vi "test5-ChainNodeBroadcast.vi"(8 "error in (no error)":errorcluster, 11 "TestCase in":refnum<class "testcase-CSMChainMode.lvclass">) -> (0 "error out":errorcluster, 3 "TestCase out":refnum<class "testcase-CSMChainMode.lvclass">)   [LabVIEW 2017, in "testcase-CSMChainMode.lvclass"]
uses:
  testcase-CSMChainMode.lvclass
  b9a68168-9423-447a-be7f-8ac0ebad77aa.vi
  a50093c0-808a-49cf-b933-7f76f8d4e341.vi
  src/user.lib/_NEVSTOP/Communicable State Machine(CSM)/AdvanceAPI/CSM - Get Module Attribute.vi
  <vilib>/addons/_JKI Toolkits/VI Tester/TestCase.llb/TestCase.lvclass
  src/user.lib/_NEVSTOP/Communicable State Machine(CSM)/Communicable State Machine.lvlib
  C:/Program Files (x86)/National Instruments/LabVIEW 2017/vi.lib/addons/_JKI Toolkits/VI Tester/TestCase.llb/TestCase.lvclass
panel:
  out "LoopCount":i32
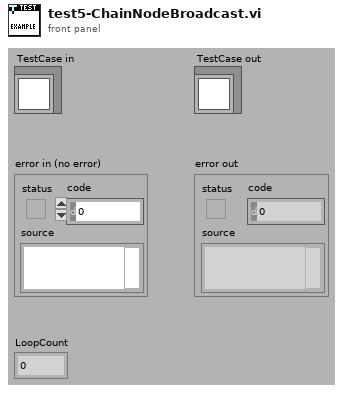
[diagram p1: front panel]
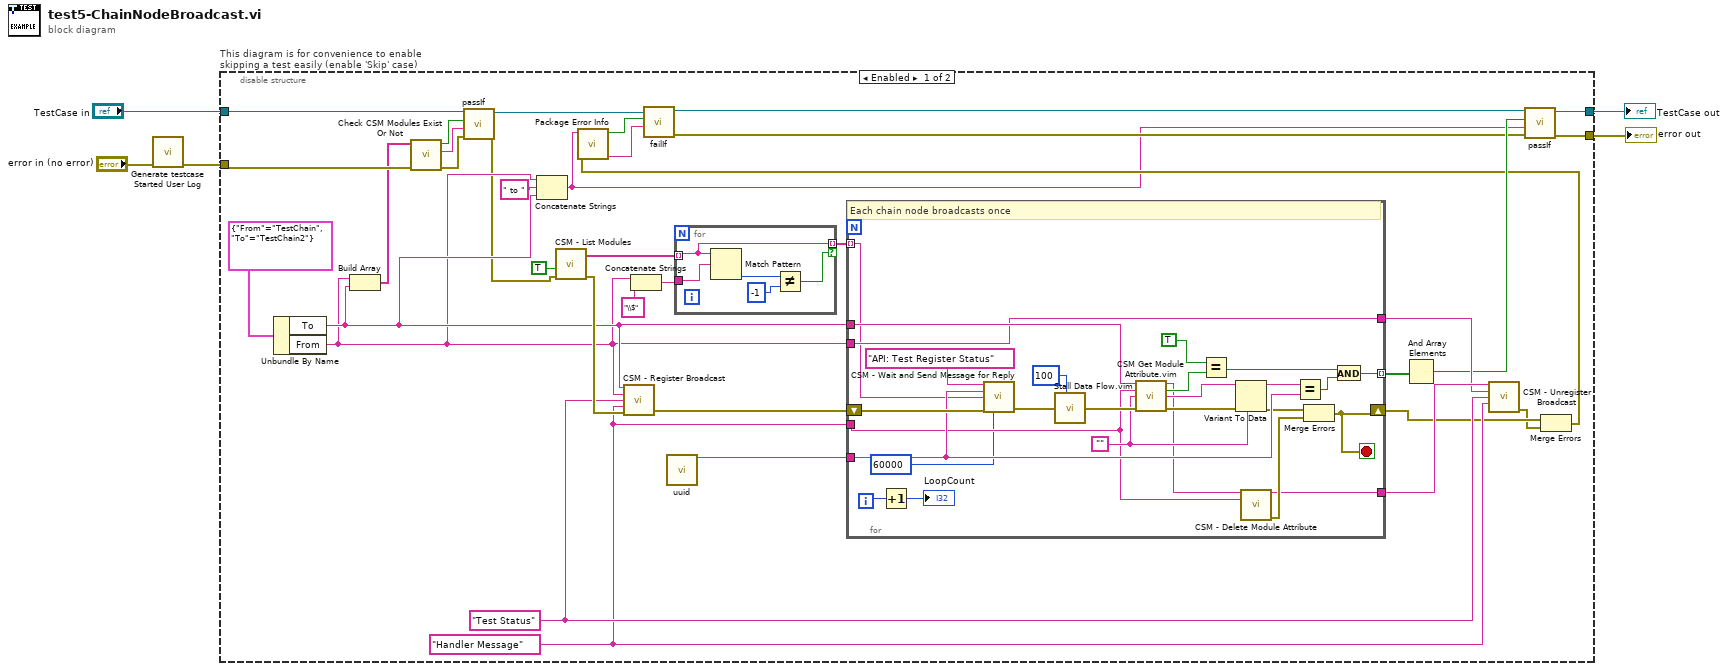
[diagram p0: block diagram]
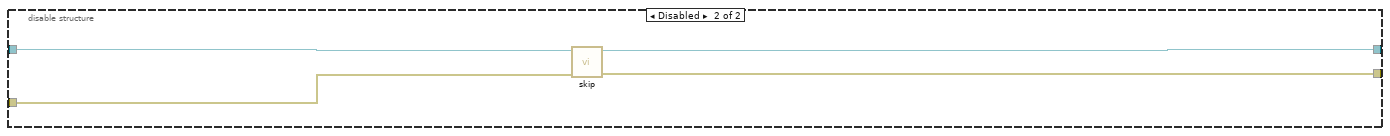
[diagram p2: hidden frame]
diagram:
  n1 = call "Generate testcase Started User Log.vi"("Error In"="error in (no error)") -> ("error out"=w1:errorcluster)  [unwired: 10 in]
  n2 = disable-structure "This diagram is for convenience to enable skipping a test easily (enable 'Skip' case)" shown="Enabled" {
    disable-tunnel: "TestCase in" -> [w15 w77]
    disable-tunnel: [w25 w75] -> w2
    disable-tunnel: [w24 w76] -> w4
    disable-tunnel: w1 -> [w13 w74]
    frame Enabled {
      w31 = "Handler Message" ("API (If \"\", Same as Trigger)")
      w32 = "Test Status" ("Trigger")
      n3 = Unbundle By Name(cluster{"From":string, "To":string} {"From"="TestChain", "To"="TestChain2"} ("Cluster")) -> ("To"=w11:string, "From"=w10:string)
      n4 = Build Array(w10, w11) -> (w12:string[])
      n5 = call "Check CSM Modules Exist Or Not.vi"("error in"=w13, "CSM names in"=w12) -> ("error out"=w20:errorcluster, "Debug string"=w21:string, "All Modules Exist?"=w22:bool)  [unwired: 7 in]
      n6 = call-dynamic "passIf.vi"("error in (no error)"=w20, "message (\"\")"=w21, "pass"=w22, "TestCase in"=w15) -> ("error out"=w9:errorcluster, "TestCase out"=w16:refnum<class "testcase-CSMChainMode.lvclass">)  [unwired: 6 in]
      n7 = Concatenate Strings(w10, " to " ("string"), w11) -> (w6:string)
      n8 = call "CSM - List Modules.vi"("Error In"=w9, "With Nodes? (F)"=TRUE) -> ("error out"=w34:errorcluster, "Module Names"=w37:string[])  [unwired: 8 in]
      n9 = call "CSM - Register Broadcast.vi"("CSM Name(Empty for Broadcast Event)"=w11, "Source CSM Name (* as Default)"=w10, "Trigger"=w32, "API (If \"\", Same as Trigger)"=w31, "Error In"=w34) -> ("error out"=w36:errorcluster)  [unwired: 9 in, 1 out]
      n10 = Concatenate Strings(w10, "\\$" ("string")) -> (w39:string)
      n11 = call "uuid.vi"() -> ("UUID"=w35:string)  [unwired: 11 in]
      n12 = for {
        tunnel: w37 -> [w71] mode=indexing
        tunnel: [w71] -> w33 mode=indexing if=w70
        tunnel: w39 -> [w69]
        n13 = Match Pattern(string=w71, regular expression=w69) -> (offset past match=w73:i32)  [unwired: 1 in, 3 out]
        n14 = Not Equal?(x=w73, y=-1) -> (x != y?=w70:bool)
      }
      n15 = for {
        tunnel: w35 -> [w54]
        tunnel: w33 -> [w44] mode=indexing
        tunnel: w11 -> [w61]
        tunnel: w31 -> [w50]
        shift-right: [w43] -> w28
        shift-left: w36 -> [w67]
        tunnel: w10 -> [w45]
        tunnel: [w47] -> w30
        tunnel: [w45] -> w29
        tunnel: [w46] -> w26 mode=indexing
        i -> [w66]
        stop <- w43 stop-if-true
        w56 = ""
        # "Each chain node broadcasts once"
        n16 = Increment(x=w66) -> (x+1=→"LoopCount":i32)
        n17 = call "CSM - Wait and Send Message for Reply.vi"("State"="API: Test Register Status", "Arguments (\"\")"=w54, "Target Module"=w44, "Error In (No Error)"=w67, "Response Timeout (-2 Using Global Settings)"=60000) -> ("error out"=w64:errorcluster)  [unwired: 7 in, 3 out]
        n18 = call "Stall Data Flow.vim"("value in"=w64, "milliseconds to wait"=u32 100) -> ("value out"=w62:errorcluster)  [unwired: 1 out]
        n19 = call "CSM Get Module Attribute.vim"("CSM Name"=w61, "Attribute"=w50, "Default Value (Empty Variant)"=w56, "Error In"=w62) -> ("CSM Name (Dup)"=w51:string, "Found"=w59:bool, "Value"=w57:string, "error out"=w58:errorcluster)  [unwired: 7 in, 1 out]
        n20 = Equal?(x=TRUE, y=w59) -> (x = y?=w52:bool)
        n21 = Variant To Data(error in=w58, type=w56, Variant=w57) -> (data=w55:string, error out=w49:errorcluster)
        n22 = call "CSM - Delete Module Attribute.vi"("CSM Name"=w51, "Attribute"=w50) -> ("CSM Name (Dup)"=w47:string, "error out"=w48:errorcluster)  [unwired: 10 in, 2 out]
        n23 = Equal?(x=w55, y=w54) -> (x = y?=w53:bool)
        n24 = Merge Errors(w49, w48) -> (w43:errorcluster)
        n25 = And(x=w52, y=w53) -> (x .and. y?=w46:bool)
      }
      n26 = And Array Elements(Boolean array=w26) -> (logical AND=w23:bool)
      n27 = call "CSM - Unregister Broadcast.vi"("CSM Name(Empty for Broadcast Event)"=w30, "Source CSM Name (* as Default)"=w29, "Trigger"=w32, "API (\"*\" as Default)"=w31) -> ("error out"=w27:errorcluster)  [unwired: 10 in, 1 out]
      n28 = Merge Errors(w28, w27) -> (w8:errorcluster)
      n29 = call "Package Error Info.vi"("error in"=w8, "String in"=w6) -> ("packed error info out"=w18:string, "error status"=w19:bool)  [unwired: 8 in]
      n30 = call-dynamic "failIf.vi"("message (\"\")"=w18, "fail"=w19, "TestCase in"=w16) -> ("error out"=w7:errorcluster, "TestCase out"=w14:refnum<class "testcase-CSMChainMode.lvclass">)  [unwired: 7 in]
      n31 = call-dynamic "passIf.vi"("error in (no error)"=w7, "message (\"\")"=w6, "pass"=w23, "TestCase in"=w14) -> ("error out"=w24:errorcluster, "TestCase out"=w25:refnum<class "testcase-CSMChainMode.lvclass">)  [unwired: 6 in]
    }
    frame Disabled {
      # "skip test result while test is under development"
      n32 = call <vilib>:"skip.vi"("error in (no error)"=w74, "TestCase in"=w77) -> ("error out"=w76:errorcluster, "TestCase out"=w75:refnum<class "testcase-CSMChainMode.lvclass">)  [unwired: 8 in]
    }
  }
  "error out" <- w4
  "TestCase out" <- w2
